vi "Get Instrument ID.vi"(4 "Check Parameters":T1={"Instrument"="Instrument", "ID Test String"="", "Terminator Character"="", "wait (mS)"=0, "Wait For SRQ"=FALSE}, 5 "Check ID":bool, 7 "VISA resource name":refnum<visa-resource-name>) -> (0 "Error Out":errorcluster {"code" format="%.0x"}, 1 "Instrument ID":string, 3 "VISA resource name":refnum<visa-resource-name>)   [LabVIEW 2019]
doc: "This VI reads the device ID string using the SCPI command *IDN?. It also attempts to detect if a listener is on the GPIB bus at that address.\nScott Hannahs, <sth@magnet.fsu.edu> NHMFL-FSU, May 2003"
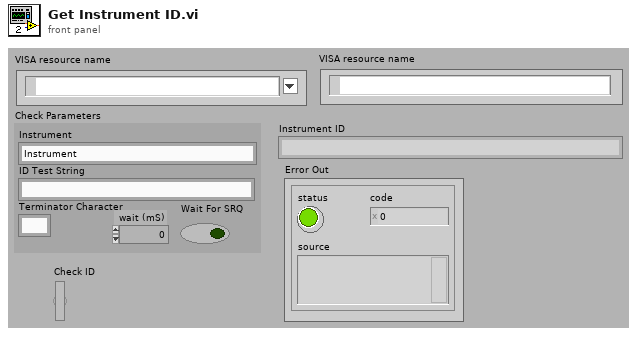
[diagram p1: front panel]
types:
  T1 = cluster{"Instrument":string, "ID Test String":string, "Terminator Character":string, "wait (mS)":u32, "Wait For SRQ":bool}
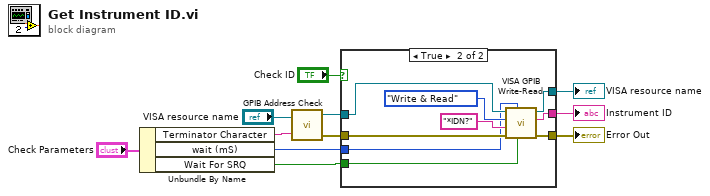
[diagram p0: block diagram]
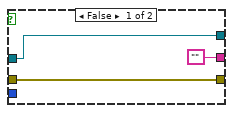
[diagram p2: hidden frame]
diagram:
  n1 = Unbundle By Name("Check Parameters") -> ("Terminator Character"=w3:string, "wait (mS)"=w2:u32, "Wait For SRQ"=w1:bool)
  n2 = call "GPIB Address Check.vi"("Instrument Address"="VISA resource name", "Term Char"=w3) -> ("dup VISA session"=w8:refnum<visa-resource-name>, "error out"=w7:errorcluster)  [unwired: 1 out]
  n3 = case shown="True" "Check ID" {
    tunnel: [w14 w23] -> w11
    tunnel: [w12 w22] -> w10
    tunnel: ["" w20] -> w9
    tunnel: w8 -> [w14 w18]
    tunnel: w7 -> [w12 w17]
    tunnel: w2 -> [_ w15]
    tunnel: w1 -> [_ w16]
    frame False {
    }
    frame True {
      n4 = call "VISA GPIB Write-Read.vi"("Wait For SRQ"=w16, "Wait (ms)"=w15, "error in (no error)"=w17, "Command"="*IDN?" ("String to Write"), "Action"=enum16{"Write", "Read", "Write & Read"}."Write & Read", "VISA resource name"=w18) -> ("error out"=w22:errorcluster, "String Returned"=w20:string, "dup VISA Session"=w23:refnum<visa-resource-name>)  [unwired: 2 in, 1 out]
    }
  }
  "VISA resource name" <- w11
  "Error Out" <- w10
  "Instrument ID" <- w9
